vi "Pre Launch Init.vi"(11 "CS++BaseActor in":refnum<class "CS++BaseActor.lvclass">) -> (0 "error out":errorcluster, 3 "CS++BaseActor out":refnum<class "CS++BaseActor.lvclass">)   [LabVIEW 2012, in "CS++BaseActor.lvlib" / "CS++BaseActor.lvclass"]
doc: "(<B>Filename</B>: Actor Framework.lvlib:Actor.lvclass:Pre Launch Init.vi)\n\nDefines behavior that occurs after the Launch Actor method is invoked but before the actor's Actor Core method begins running.\n\nThe Pre Launch Init method is guaranteed to finish before the Launch Actor method returns to its caller and before the actor itself receives any messages. Any references that the Pre Launch Init method obtains are guaranteed to have the same lifetime as the actor itself. Any errors that the Pre Launch Init method returns will abort the launch.\n\nBy default, this method does nothing. A descendant class may override it to define behavior."
uses:
  CS++BaseActor.lvclass
  <vilib>/ActorFramework/Actor/Actor.lvclass
  CS++BaseActor.lvclass/CS++BaseActor.ctl
  Libraries/MessageLogger/CS++MessageLogger.lvlib
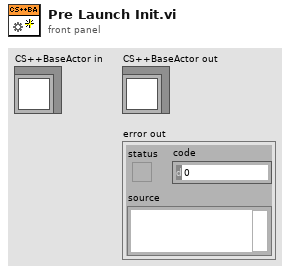
[diagram p1: front panel]
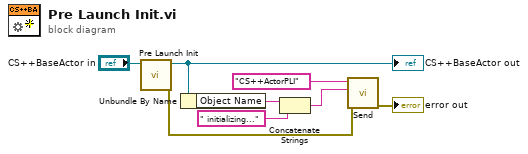
[diagram p0: block diagram]
diagram:
  n1 = call-parent "Pre Launch Init.vi"("Actor in"="CS++BaseActor in") -> ("error out"=w2:errorcluster, "Actor out"=w7:refnum<class "CS++BaseActor.lvclass">)  [unwired: 9 in]
  "CS++BaseActor out" <- w7
  n2 = Unbundle By Name(w7) -> ("Object Name"=w4:string)
  n3 = Concatenate Strings(w4, " initializing..." ("string")) -> (w5:string)
  n4 = call "Send.vi"("Error In"=w2, "Message Content"=w5, "Message Tag"="CS++ActorPLI") -> ("Error Out"=→"error out":errorcluster)  [unwired: 8 in]
